vi "Configure Digital Input Attenuation Level.vi"(8 "error in (no error)":errorcluster, 9 "Input Attenuation Level (50.000 mV)":dbl=50.0 format="%.8e", 10 "Input Attenuation Mode (0: Default)":i32(ring) items=["Default", "Manual"], 11 "VISA resource name":refnum<visa-resource-name>) -> (0 "error out":errorcluster, 3 "VISA resource name out":refnum<visa-resource-name>)   [LabVIEW 2018, in "Agilent PSG MXG Series.lvlib"]
doc: "Configures the digital input attenuation level.\n\n<b>Note:</b>\nIt is applicable for N5172B/82B with <b>Option 004</b> only."
uses:
  Agilent PSG MXG Series.lvlib
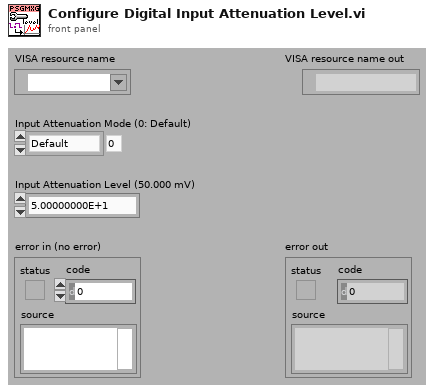
[diagram p1: front panel]
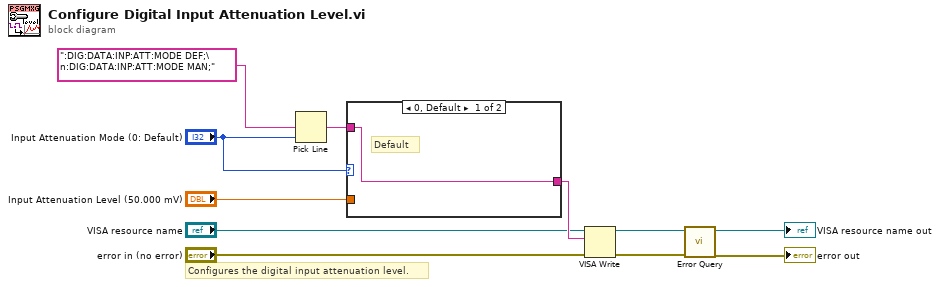
[diagram p0: block diagram]
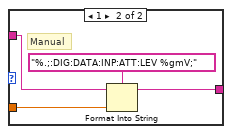
[diagram p2: hidden frame]
diagram:
  # "Configures the digital input attenuation level."
  n1 = Pick Line(multi-line string=":DIG:DATA:INP:ATT:MODE DEF;\n:DIG:DATA:INP:ATT:MODE MAN;", line index="Input Attenuation Mode (0: Default)") -> (output string=w1:string)  [unwired: 1 in]
  n2 = case shown="0, Default" "Input Attenuation Mode (0: Default)" {
    tunnel: "Input Attenuation Level (50.000 mV)" -> [_ w15]
    tunnel: [w12 w14] -> w10
    tunnel: w1 -> [w12 w13]
    frame 0, Default {
      # "Default"
    }
    frame 1 {
      # "Manual"
      n3 = Format Into String(format string="%.;:DIG:DATA:INP:ATT:LEV %gmV;", initial string=w13, w15) -> (resulting string=w14:string)  [unwired: 1 in, 1 out]
    }
  }
  n4 = VISA Write(VISA resource name="VISA resource name", write buffer=w10, error in (no error)="error in (no error)") -> (VISA resource name out=w7:refnum<visa-resource-name>, error out=w6:errorcluster)  [unwired: 1 out]
  n5 = call "Error Query.vi"("error in (no error)"=w6, "VISA resource name"=w7) -> ("error out"=→"error out":errorcluster, "VISA resource name out"=→"VISA resource name out":refnum<visa-resource-name>)  [unwired: 6 in, 2 out]
